vi "17.ShapeRecognition.vi"() -> ()   [LabVIEW 2017]
uses:
  <vilib>/userdefined/High Color/IMAQdx.ctl
  <vilib>/vision/driver/NI_Vision_Acquisition_Software.lvlib
  <vilib>/vision/NI_Vision_Development_Module.lvlib
panel:
  out "检测到圆形":bool
  out "Circles Data":T1(array[cluster])
  out "Image Out":T2(plugin-control)
  out "error out":errorcluster
  out "Image Hull":T2(plugin-control)
  out "Image Filter":T2(plugin-control)
  out "Image Threshold":T2(plugin-control)
  out "Image In":T2(plugin-control)
  in  "停止":bool
  in  "Camera Select":T3
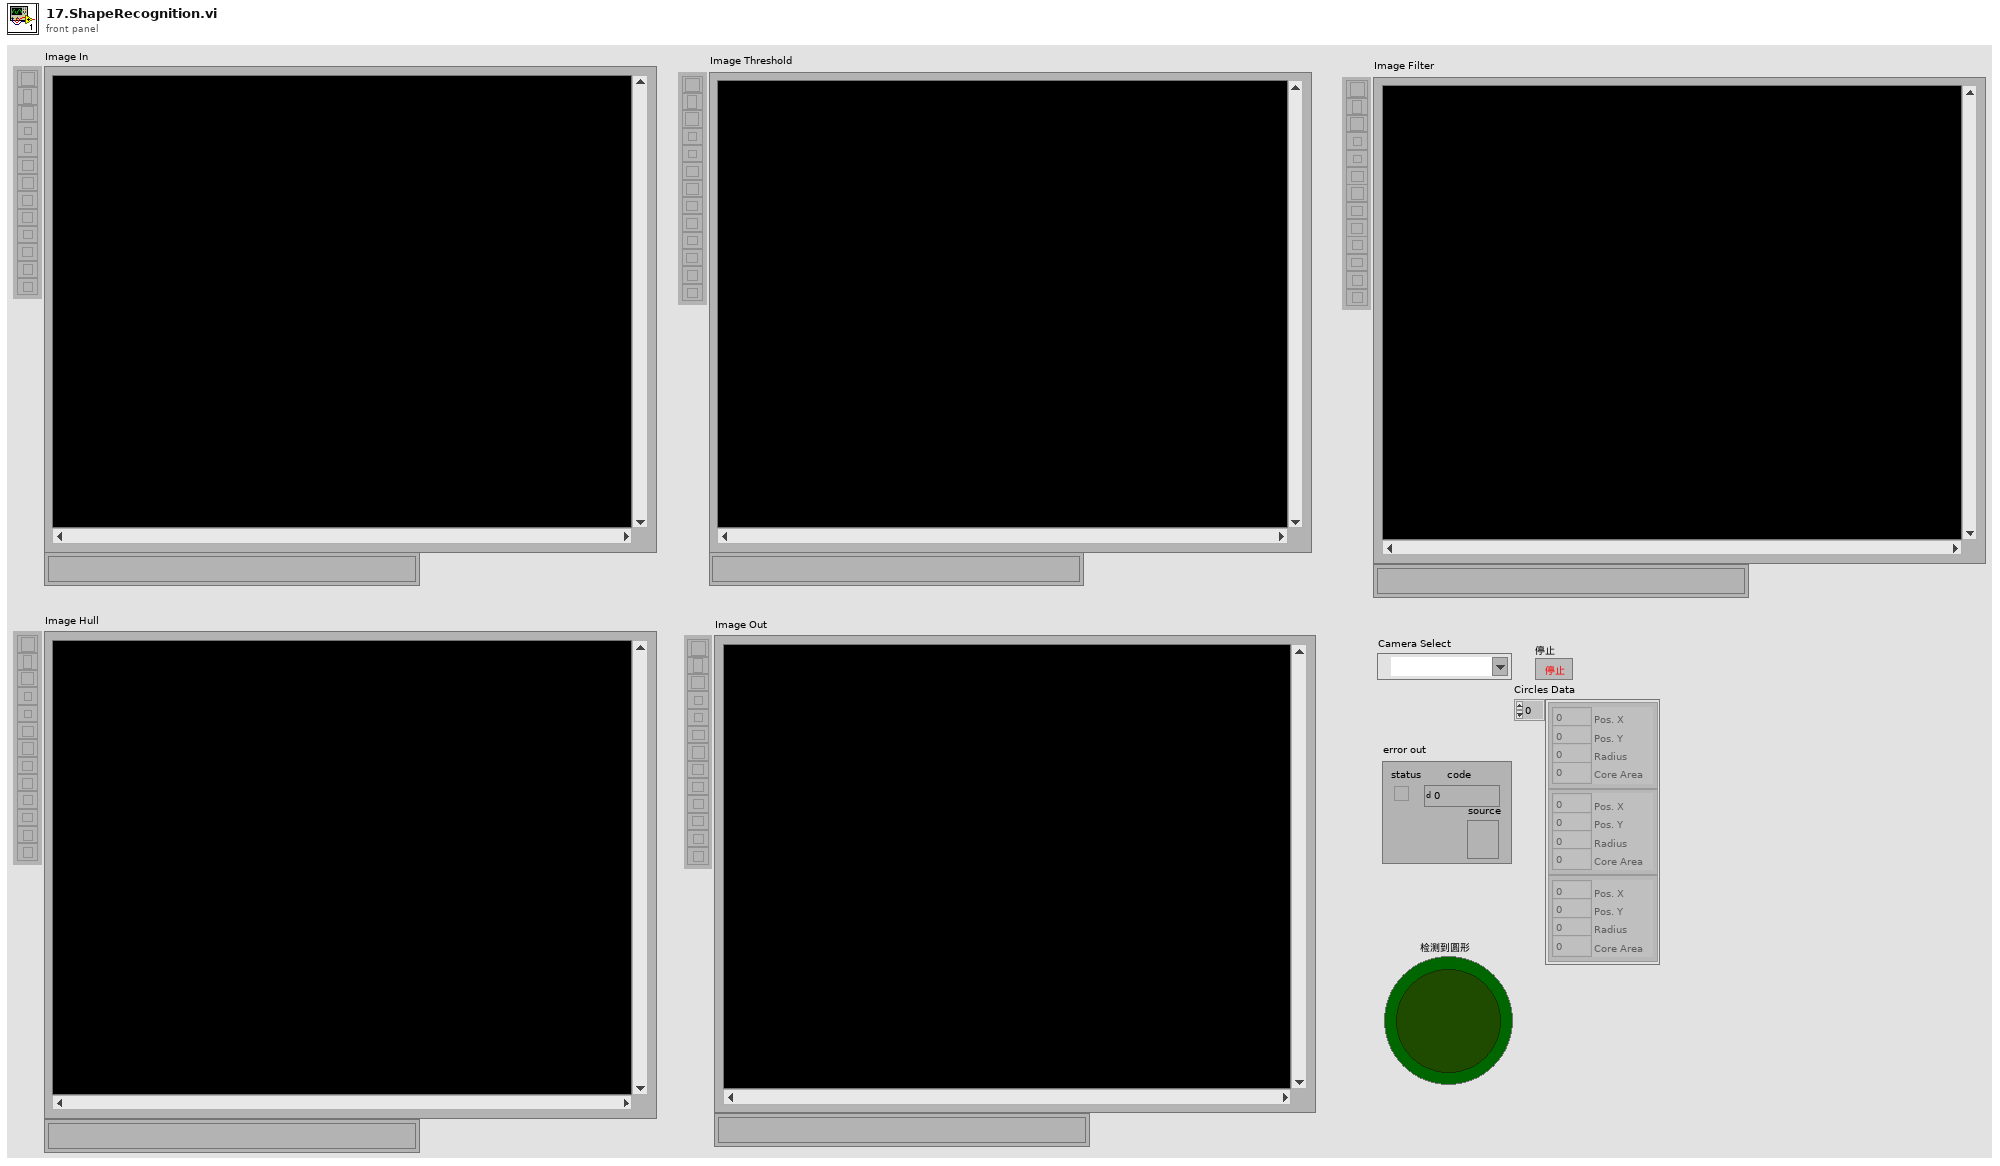
[diagram p1: front panel]
types:
  T1 = cluster{"Pos. X":i32, "Pos. Y":i32, "Radius":i32, "Core Area":i32}[]
  T2 = typedef "IMAQ Image.ctl" = refnum<image>
  T3 = typedef "IMAQdx.ctl" = refnum<k21>
  T4 = cluster{"Global Rectangle":i32[], "Contours":cluster{"ID":enum32{"External", "Internal"}, "Type":u32, "Coordinates":i32[]}[]}
  T5 = cluster{"Pos. X":i32, "Pos. Y":i32, "Radius":i32, "Core Area":i32}
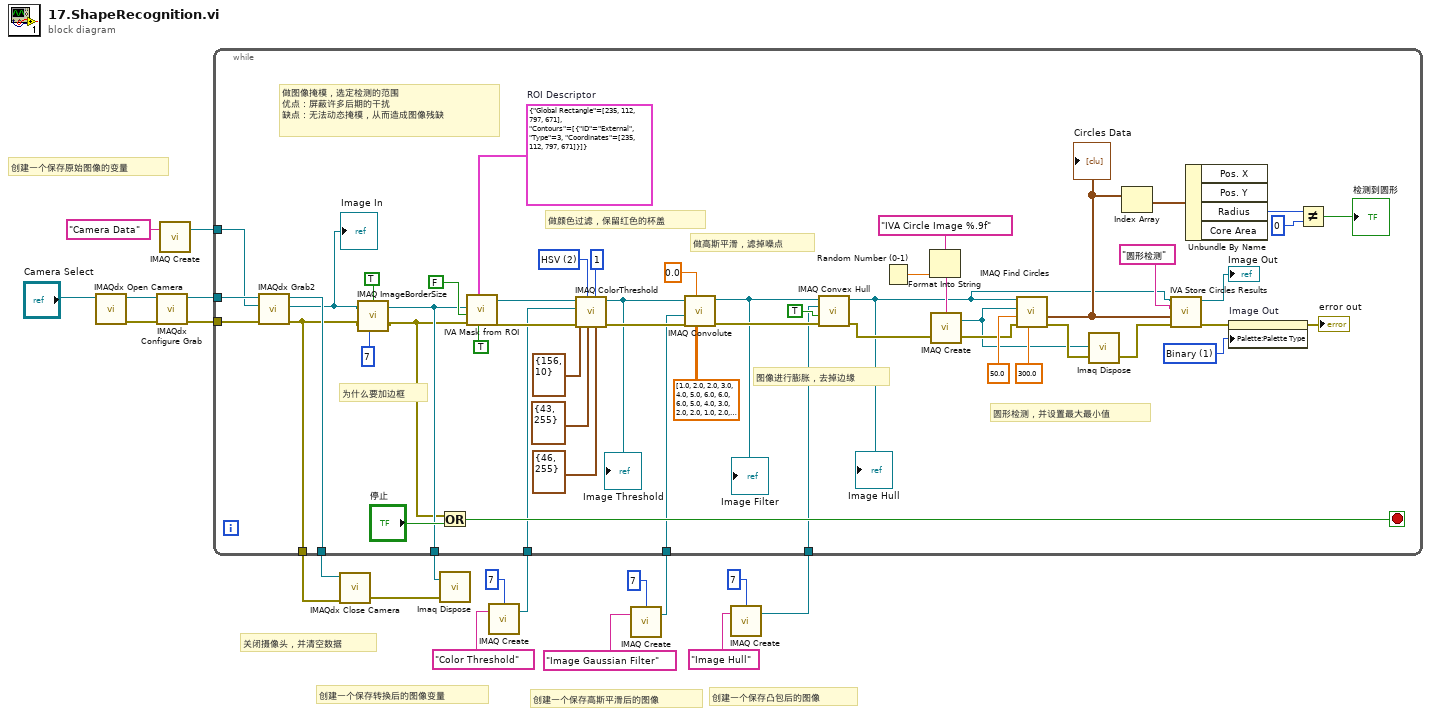
[diagram p0: block diagram]
diagram:
  # "创建一个保存凸包后的图像"
  # "创建一个保存高斯平滑后的图像"
  # "创建一个保存原始图像的变量"
  # "创建一个保存转换后的图像变量"
  # "关闭摄像头，并清空数据"
  n1 = call <vilib>:"IMAQdx Open Camera.vi"("Session In"="Camera Select") -> ("error out"=w20:errorcluster, "Session Out"=w19:T3)  [unwired: 9 in]
  n2 = call <vilib>:"IMAQdx Configure Grab.vi"("error in"=w20, "Session In"=w19) -> ("error out"=w17:errorcluster, "Session Out"=w18:T3)  [unwired: 8 in]
  n3 = call "IMAQ Create"("Image Name"="Camera Data") -> ("New Image"=w16:T2)  [unwired: 4 in, 1 out]
  n4 = call "IMAQ Create"("Border Size"=7, "Image Name"="Color Threshold") -> ("New Image"=w9:T2)  [unwired: 3 in, 1 out]
  n5 = call "IMAQ Create"("Border Size"=7, "Image Name"="Image Gaussian Filter") -> ("New Image"=w4:T2)  [unwired: 3 in, 1 out]
  n6 = call "IMAQ Create"("Border Size"=7, "Image Name"="Image Hull") -> ("New Image"=w1:T2)  [unwired: 3 in, 1 out]
  n7 = while {
    tunnel: w18 -> [w73]
    tunnel: w17 -> [w72]
    tunnel: w16 -> [w71]
    tunnel: [w52] -> w13
    tunnel: [w49] -> w12
    tunnel: [w50] -> w10
    tunnel: w9 -> [w53]
    tunnel: w4 -> [w43]
    tunnel: w1 -> [w42]
    stop <- w61 stop-if-true
    w37 = u32 1 items=["Grayscale", "Binary", "Gradient", "Rainbow", "Temperature", "User Defined", "Binary 16 Bit", "Gradient 16 Bit", "Rainbow 16 Bit", "Temperature 16 Bit", "User Defined 16 Bit"] ("Palette Type")
    w66 = u16 2 items=["RGB", "HSL", "HSV", "HSI"] ("Color Mode")
    w70 = T4 {"Global Rectangle"=[235, 112, 797, 671], "Contours"=[{"ID"=enum."External", "Type"=3, "Coordinates"=[235, 112, 797, 671]}]}  # ROI Descriptor
    # "圆形检测，并设置最大最小值"
    # "为什么要加边框"
    # "图像进行膨胀，去掉边缘"
    # "做高斯平滑，滤掉噪点"
    # "做颜色过滤，保留红色的杯盖"
    # "做图像掩模，选定检测的范围\n优点：屏蔽许多后期的干扰\n缺点：无法动态掩模，从而造成图像残缺"
    n8 = call <vilib>:"IMAQdx Grab2.vi"("error in"=w72, "Image In"=w71, "Session In"=w73) -> ("error out"=w49:errorcluster, "Image Out"=w51:T2, "Session Out"=w52:T3)  [unwired: 5 in, 1 out]
    "Image In" <- w51
    n9 = call "IMAQ ImageBorderSize"("Get/Set Status? (Set)"=TRUE, "Image"=w51, "Image border size in"=7, "error in (no error)"=w49) -> ("Image Out"=w50:T2, "error out"=w48:errorcluster)  [unwired: 1 out]
    n10 = Or(x=w48, y="停止") -> (x .or. y?=w61:bool)
    n11 = call <vilib>:"IVA Mask from ROI.vi"("Shrink"=TRUE, "ROI Descriptor"=w70, "error in (no error)"=w48, "Out / In"=FALSE, "Image Src"=w50) -> ("error out"=w62:errorcluster, "Image Out"=w58:T2)  [unwired: 5 out]
    n12 = call "IMAQ ColorThreshold"("Blue or Luma or Val or Inten Range"=cluster{"Lower value":i32, "Upper value":i32} {"Lower value"=46, "Upper value"=255}, "Replace Value"=1, "Green or Sat Range"=cluster{"Lower value":i32, "Upper value":i32} {"Lower value"=43, "Upper value"=255}, "Color Mode"=w66, "error in (no error)"=w62, "Red or Hue Range"=cluster{"Lower value":i32, "Upper value":i32} {"Lower value"=156, "Upper value"=10}, "Image Dst"=w53, "Image Src"=w58) -> ("error out"=w57:errorcluster, "Image Dst Out"=w45:T2)  [unwired: 2 out]
    "Image Threshold" <- w45
    n13 = call "IMAQ Convolute"("Kernel"=sgl[][] [[1.0, 2.0, 2.0, 3.0, 4.0, 5.0, 6.0, 6.0, 6.0, 5.0, 4.0, 3.0, 2.0, 2.0, 1.0], [2.0, 3.0, 4.0, 5.0, 7.0, 8.0, 9.0, 9.0, 9.0, 8.0, 7.0, 5.0, 4.0, 3.0, 2.0], [2.0, 4.0, 6.0, 8.0, 10.0, 12.0, 13.0, 13.0, 13.0, 12.0, 10.0, 8.0, 6.0, 4.0, 2.0], [3.0, 5.0, 8.0, 10.0, 13.0, 16.0, 18.0, 18.0, 18.0, 16.0, 13.0, 10.0, 8.0, 5.0, 3.0], [4.0, 7.0, 10.0, 13.0, 17.0, 21.0, 23.0, 24.0, 23.0, 21.0, 17.0, 13.0, 10.0, 7.0, 4.0], [5.0, 8.0, 12.0, 16.0, 21.0, 25.0, 27.0, 28.0, 27.0, 25.0, 21.0, 16.0, 12.0, 8.0, 5.0], [6.0, 9.0, 13.0, 18.0, 23.0, 27.0, 30.0, 31.0, 30.0, 27.0, 23.0, 18.0, 13.0, 9.0, 6.0], [6.0, 9.0, 13.0, 18.0, 24.0, 28.0, 31.0, 33.0, 31.0, 28.0, 24.0, 18.0, 13.0, 9.0, 6.0], [6.0, 9.0, 13.0, 18.0, 23.0, 27.0, 30.0, 31.0, 30.0, 27.0, 23.0, 18.0, 13.0, 9.0, 6.0], [5.0, 8.0, 12.0, 16.0, 21.0, 25.0, 27.0, 28.0, 27.0, 25.0, 21.0, 16.0, 12.0, 8.0, 5.0], [4.0, 7.0, 10.0, 13.0, 17.0, 21.0, 23.0, 24.0, 23.0, 21.0, 17.0, 13.0, 10.0, 7.0, 4.0], [3.0, 5.0, 8.0, 10.0, 13.0, 16.0, 18.0, 18.0, 18.0, 16.0, 13.0, 10.0, 8.0, 5.0, 3.0], [2.0, 4.0, 6.0, 8.0, 10.0, 12.0, 13.0, 13.0, 13.0, 12.0, 10.0, 8.0, 6.0, 4.0, 2.0], [2.0, 3.0, 4.0, 5.0, 7.0, 8.0, 9.0, 9.0, 9.0, 8.0, 7.0, 5.0, 4.0, 3.0, 2.0], [1.0, 2.0, 2.0, 3.0, 4.0, 5.0, 6.0, 6.0, 6.0, 5.0, 4.0, 3.0, 2.0, 2.0, 1.0]], "Divider (kernel sum)"=sgl 0.0 ("Divider"), "error in (no error)"=w57, "Image Dst"=w43, "Image Src"=w45) -> ("error out"=w56:errorcluster, "Image Dst Out"=w44:T2)  [unwired: 2 in, 3 out]
    "Image Filter" <- w44
    n14 = call "IMAQ Convex Hull"("error in (no error)"=w56, "Connectivity 4/8 (8)"=TRUE, "Image Dst"=w42, "Image Src"=w44) -> ("error out"=w31:errorcluster, "Image Dst Out"=w21:T2)  [unwired: 6 out]
    "Image Hull" <- w21
    n15 = Random Number (0-1)() -> (number: 0 to 1=w34:dbl)
    n16 = Format Into String(format string="IVA Circle Image %.9f" ("格式字符串"), w34) -> (resulting string=w33:string)  [unwired: 2 in, 1 out]
    n17 = call "IMAQ Create"("Image Name"=w33, "error in (no error)"=w31) -> ("New Image"=w27:T2, "error out"=w30:errorcluster)  [unwired: 3 in]
    n18 = call "IMAQ Find Circles"("Max Radius"=sgl 300.0, "error in (no error)"=w30, "Min Radius"=sgl 50.0, "Image Dst"=w27, "Image Src"=w21) -> ("error out"=w29:errorcluster, "Circles Data"=w26:T1)  [unwired: 5 out]
    "Circles Data" <- w26
    n19 = call "Imaq Dispose"("Image"=w27, "error in (no error)"=w29) -> ("error out"=w28:errorcluster)  [unwired: 4 in]
    n20 = Index Array(array=w26) -> (element=w25:T5)  [unwired: 1 in]
    n21 = call <vilib>:"IVA Store Circles Results.vi"("error in (no error)"=w28, "Circles Data"=w26, "Step Name"="圆形检测", "Image in"=w21) -> ("error out"=w38:errorcluster, "Image dup"=→"Image Out":T2)  [unwired: 6 out]
    n22 = Unbundle By Name(w25) -> ("Radius"=w24:i32)  [unwired: 3 out]
    n23 = property on="Image Out" class="ImageControl"(error in=w38, "Palette:Palette Type"=w37) -> (error out=→"error out":errorcluster)  [unwired: 1 in, 1 out]
    n24 = Not Equal?(x=w24, y=0) -> (x != y?=→"检测到圆形":bool)
  }
  n25 = call <vilib>:"IMAQdx Close Camera.vi"("error in"=w12, "Session In"=w13) -> ("error out"=w11:errorcluster)  [unwired: 9 in]
  n26 = call "Imaq Dispose"("Image"=w10, "error in (no error)"=w11) -> ()  [unwired: 4 in, 1 out]
